vi "Excel文件读写.vi"(0 "选项":T1, 1 "sheet name":string="ASDE", 2 "列首名称":string[](array[string]) caption="列首", 3 "表格":string[][](table), 4 "单个结果":bool[][](array[boolean]), 5 "error in":errorcluster caption="错误输入（无错误）", 6 "Path":path=path "D:/123.xls") -> (14 "表格操作正常":bool, 15 "data":string[][](table), 19 "error out":errorcluster caption="错误输出")   [LabVIEW 2014]
uses:
  <vilib>/addons/_office/excel.llb/Excel Get Data ([str]).vi
  <vilib>/Utility/NIReport.llb/Append Text Table to Report (wrap).vi
  <vilib>/Utility/NIReport.llb/NI_report.lvclass
  <vilib>/Utility/NIReport.llb/Excel/NI_Excel.lvclass
  <vilib>/addons/_office/NI_ReportGenerationToolkit.lvlib
panel:
  out "error out 2":errorcluster caption="error out"
  in  "Cpk计算数量":i32
  out "Path 2":path
  out "结束行":cluster{"row":i32, "column":i32}
  out "起始":cluster{i32, i32}
  out "position (Excel)":cluster{"row":i32, "column":i32}
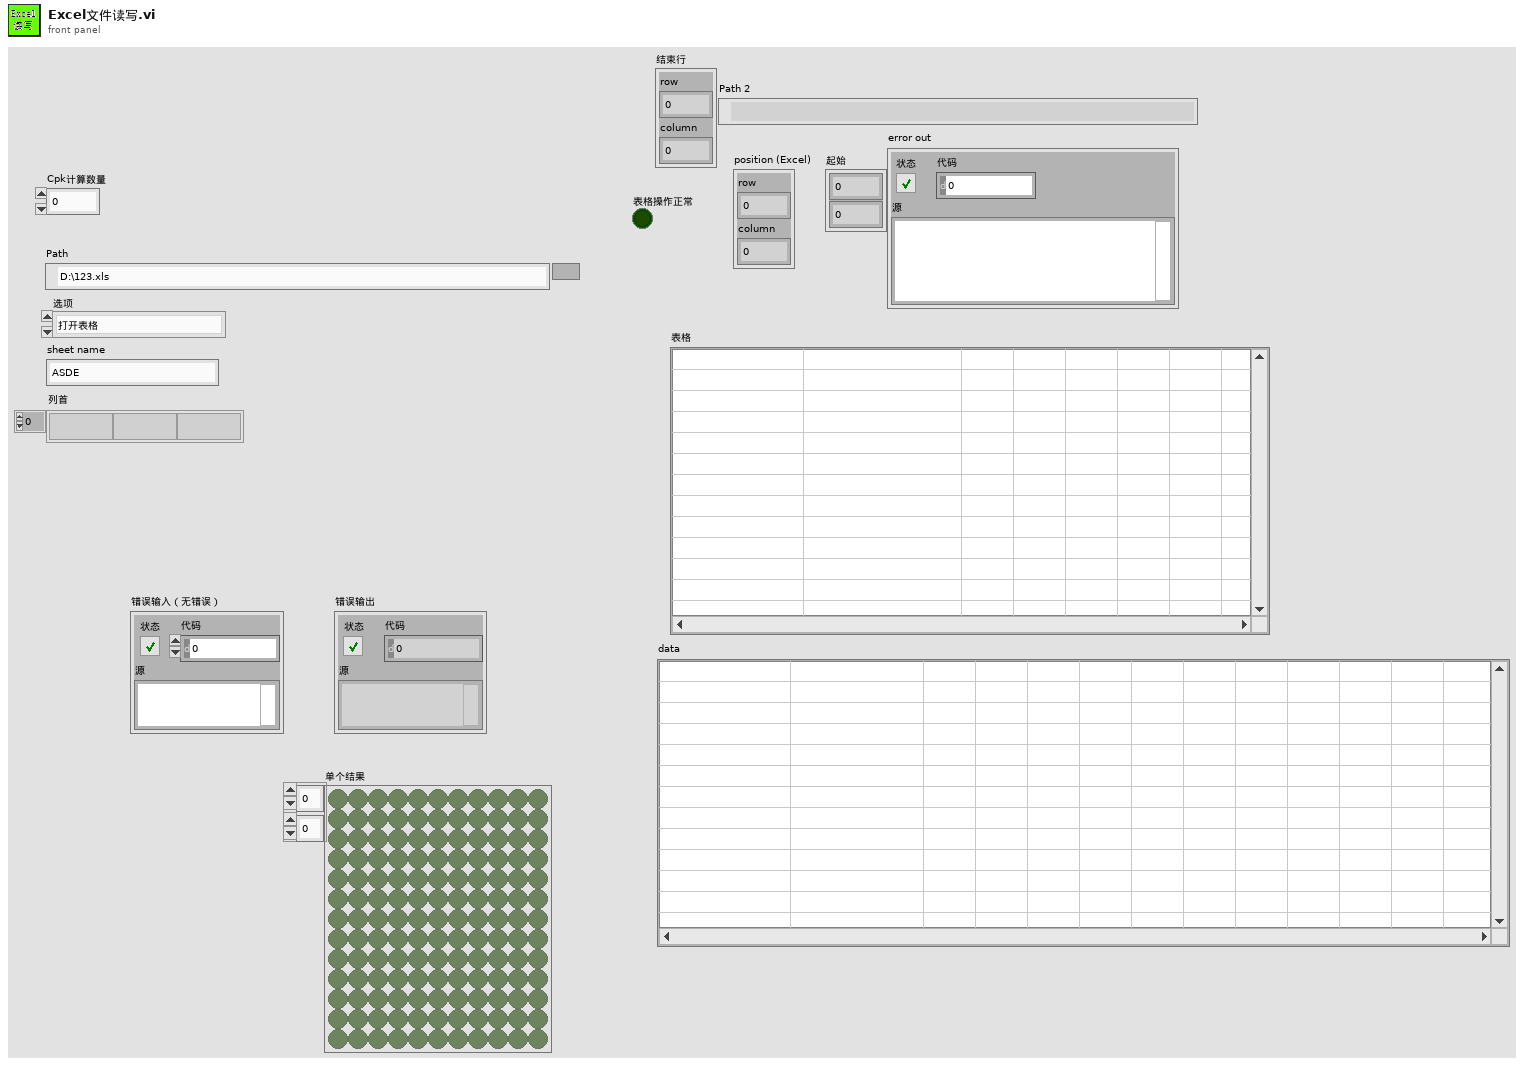
[diagram p1: front panel]
types:
  T1 = typedef "控件-Excel读写选项.ctl" = enum16{"打开表格", "新增sheet", "读取sheet指定位置数据", "读取sheet整个数据", "写入sheet整个数据", "写表头", "数据存到本机", "表格是否开启状态", "关闭表格"}
  T2 = enum16{"maximized", "minimized", "normal", "no change"}
  T3 = enum16{"Standard Report", "HTML", "Word", "Excel"}
  T4 = cluster{"position (Excel)":cluster{"row":i32, "column":i32}, "name (Excel)":string, "bookmark (Word)":string}
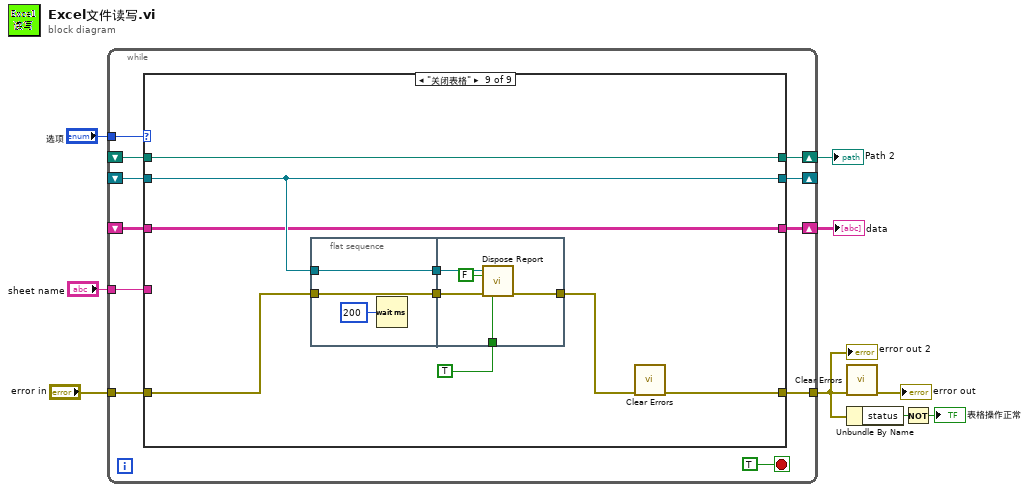
[diagram p0: block diagram]
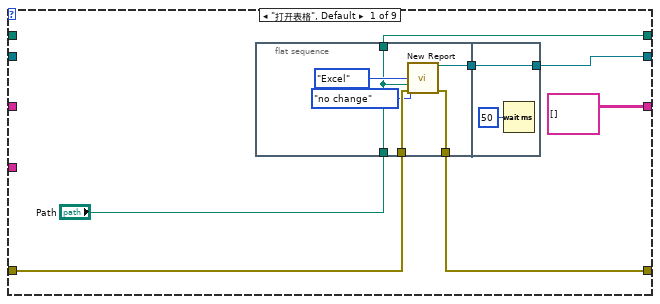
[diagram p2: hidden frame]
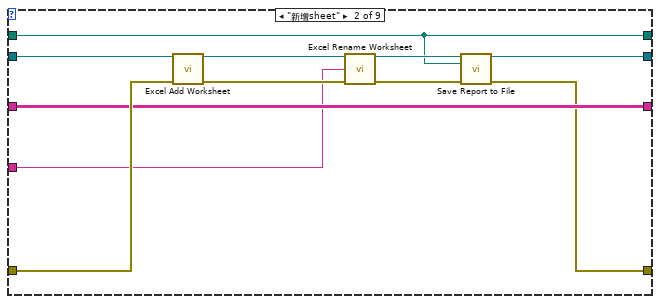
[diagram p3: hidden frame]
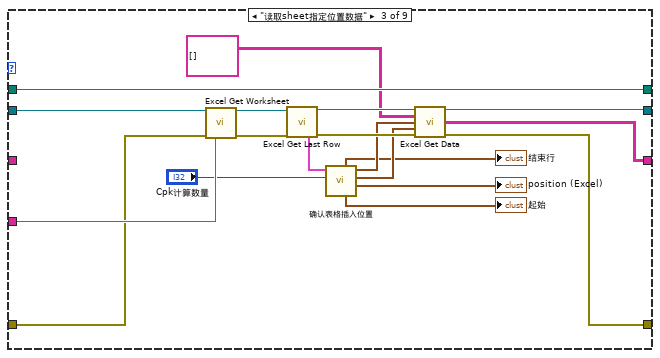
[diagram p4: hidden frame]
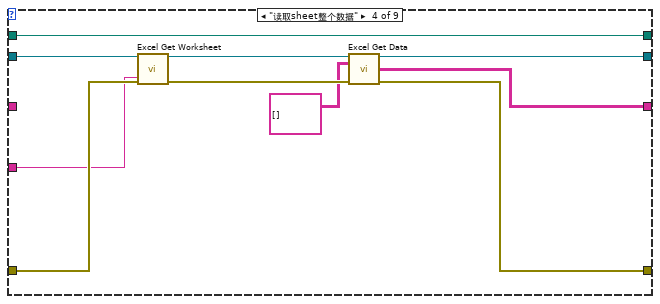
[diagram p5: hidden frame]
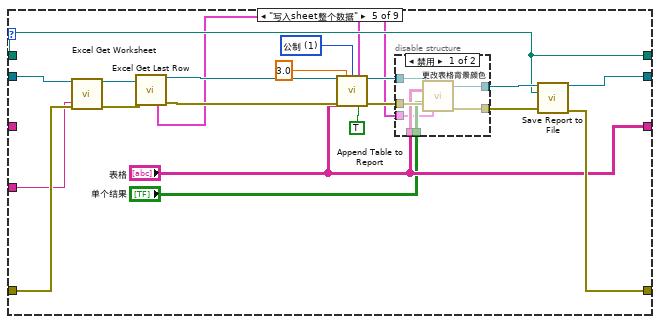
[diagram p6: hidden frame]
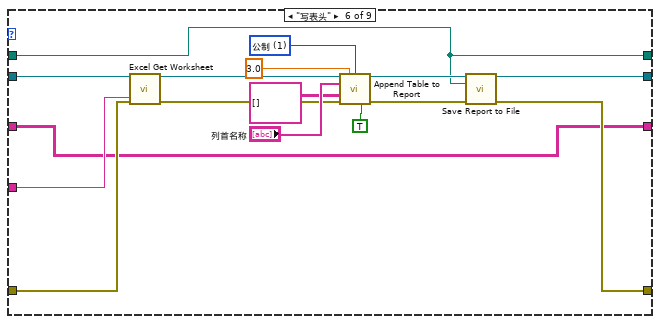
[diagram p8: hidden frame]
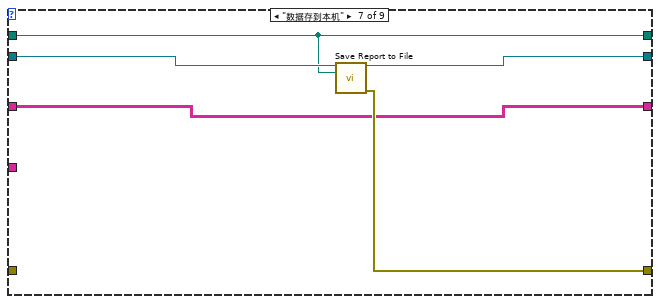
[diagram p9: hidden frame]
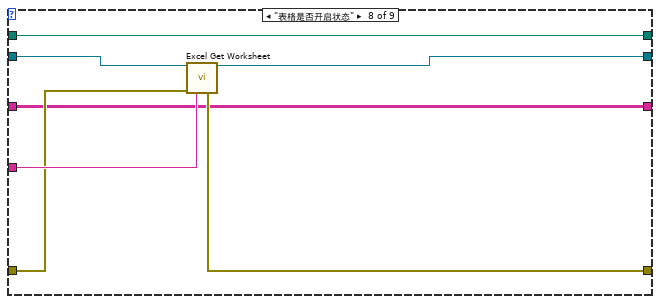
[diagram p10: hidden frame]
diagram:
  n1 = while {
    tunnel: "选项" -> [w19]
    shift-right: [w18] -> _
    shift-left: _ -> [w17]
    tunnel: "error in" -> [w16]
    tunnel: [w15] -> w4
    shift-right: [w14] -> w7
    shift-left: _ -> [w13]
    tunnel: "sheet name" -> [w12]
    shift-right: [w10] -> w1
    shift-left: _ -> [w11]
    stop <- TRUE stop-if-true
    n2 = case shown="\"关闭表格\"" w19 {
      tunnel: [w27 w39 w64 w73 w95 w115 w124 w128 w140] -> w18
      tunnel: w17 -> [_ w45 w56 w75 w90 w112 w125 w132 w140]
      tunnel: w16 -> [w26 w44 w57 w70 w89 w108 _ w130 w141]
      tunnel: [w25 w37 w65 w71 w94 w107 w123 w129 w136] -> w15
      tunnel: [string[][] [] ("data") w42 w63 w68 "表格" w105 w122 w126 w139] -> w14
      tunnel: w13 -> [_ w42 _ _ _ w105 w122 w126 w139]
      tunnel: w12 -> [_ w41 w58 w67 w88 w109 _ w131 _]
      tunnel: w11 -> [_ w36 w62 w66 w83 w110 w121 w127 w135]
      tunnel: [w22 w36 w62 w66 w83 w110 w121 w127 w135] -> w10
      frame "打开表格", Default {
        n3 = flat-sequence {
          tunnel: w26 -> [w32]
          tunnel: [w31] -> w25
          tunnel: "Path" -> [w28]
          tunnel: [w33] -> w23
          tunnel: [w28] -> w22
          tunnel: [w35] -> w27
          tunnel: w23 -> [w35]
          frame #0 {
            n4 = call <vilib>:"New Report.vi"("window state (normal)"=T2."no change", "report type"=T3."Excel", "template (empty)"=w28, "error in (no error)"=w32) -> ("report out"=w33:refnum<class "NI_report.lvclass">, "error out"=w31:errorcluster)  [unwired: 10 in]
          }
          frame #1 {
            n5 = Wait (ms)(milliseconds to wait=u32 50 ("等待时间（毫秒）")) -> ()  [unwired: 1 out]
          }
        }
      }
      frame "新增sheet" {
        n6 = call <vilib>:"Excel Add Worksheet.vi"("report in"=w45, "error in (no error)"=w44) -> ("report out"=w46:refnum<class "NI_report.lvclass">, "error out"=w43:errorcluster)  [unwired: 12 in]
        n7 = call <vilib>:"Excel Rename Worksheet.vi"("report in"=w46, "worksheet name (\"\")"=w41, "error in (no error)"=w43) -> ("report out"=w40:refnum<class "NI_report.lvclass">, "error out"=w38:errorcluster)  [unwired: 11 in]
        n8 = call-dynamic "Save Report to File.vi"("report in"=w40, "report file path"=w36, "error in (no error)"=w38) -> ("report out"=w39:refnum<class "NI_report.lvclass">, "error out"=w37:errorcluster)  [unwired: 11 in]
      }
      frame "读取sheet指定位置数据" {
        n9 = call <vilib>:"Excel Get Worksheet.vi"("report in"=w56, "error in (no error)"=w57, "name (\"\")"=w58) -> ("report out"=w55:refnum<class "NI_report.lvclass">, "error out"=w54:errorcluster)  [unwired: 11 in]
        n10 = call <vilib>:"Excel Get Last Row.vi"("report in"=w55, "error in (no error)"=w54) -> ("report out"=w61:refnum<class "NI_report.lvclass">, "MS Office parameters out"=w60:T4, "error out"=w59:errorcluster)  [unwired: 11 in]
        n11 = call "确认表格插入位置.vi"("Cpk计算数量"="Cpk计算数量", "MS Office parameters out"=w60) -> ("position (Excel)"=→"position (Excel)":cluster{"row":i32, "column":i32}, "簇"=w51:cluster{"row":i32, i32}, "簇 2"=w52:cluster{"f":i32, i32}, "起始"=→"起始":cluster{i32, i32}, "结束行"=→"结束行":cluster{"row":i32, "column":i32})  [unwired: 5 in]
        n12 = call-poly <vilib>:"Excel Get Data.vi"("report in"=w61, "data type"=string[][] [], "start (-1, -1)"=w52, "end (-1, -1)"=w51, "error in (no error)"=w59) -> ("report out"=w64:refnum<class "NI_report.lvclass">, "data"=w63:string[][], "error out"=w65:errorcluster)  [unwired: 8 in]
      }
      frame "读取sheet整个数据" {
        n13 = call <vilib>:"Excel Get Worksheet.vi"("report in"=w75, "error in (no error)"=w70, "name (\"\")"=w67) -> ("report out"=w74:refnum<class "NI_report.lvclass">, "error out"=w72:errorcluster)  [unwired: 11 in]
        n14 = call-poly <vilib>:"Excel Get Data.vi"("report in"=w74, "data type"=string[][] [], "error in (no error)"=w72) -> ("report out"=w73:refnum<class "NI_report.lvclass">, "data"=w68:string[][], "error out"=w71:errorcluster)  [unwired: 10 in]
      }
      frame "写入sheet整个数据" {
        w93 = u16 1 items=["US", "公制", "默认"] ("measurement system")
        n15 = call <vilib>:"Excel Get Worksheet.vi"("report in"=w90, "error in (no error)"=w89, "name (\"\")"=w88) -> ("report out"=w82:refnum<class "NI_report.lvclass">, "error out"=w81:errorcluster)  [unwired: 11 in]
        n16 = call <vilib>:"Excel Get Last Row.vi"("report in"=w82, "error in (no error)"=w81) -> ("report out"=w79:refnum<class "NI_report.lvclass">, "MS Office parameters out"=w76:T4, "error out"=w80:errorcluster)  [unwired: 11 in]
        n17 = call-poly <vilib>:"Append Table to Report.vi"("report in"=w79, "column width (1)"=3.0, "measurement system"=w93, "MS Office parameters"=w76, "text data"="表格", "error in (no error)"=w80, "show grid lines (YES)"=TRUE) -> ("report out"=w87:refnum<class "NI_report.lvclass">, "error out"=w85:errorcluster)  [unwired: 5 in, 2 out]
        n18 = disable-structure shown="禁用" {
          disable-tunnel: w87 -> [w102 w104]
          disable-tunnel: [w101 w103] -> w86
          disable-tunnel: w85 -> [w100 w103]
          disable-tunnel: [w99 w104] -> w84
          disable-tunnel: "表格" -> [w98 _]
          disable-tunnel: "单个结果" -> [w97 _]
          disable-tunnel: w76 -> [w96 _]
          frame Disabled {
            n19 = call "更改表格背景颜色.vi"("NI_report输入"=w102, "表格"=w98, "单个结果"=w97, "错误输入（无错误）"=w100, "MS Office parameters out"=w96) -> ("NI_report输出"=w99:refnum<class "NI_report.lvclass">, "错误输出"=w101:errorcluster)  [unwired: 9 in]
          }
          frame Enabled {
          }
        }
        n20 = call-dynamic "Save Report to File.vi"("report in"=w84, "report file path"=w83, "error in (no error)"=w86) -> ("report out"=w95:refnum<class "NI_report.lvclass">, "error out"=w94:errorcluster)  [unwired: 11 in]
      }
      frame "写表头" {
        w120 = u16 1 items=["US", "公制", "默认"] ("measurement system")
        n21 = call <vilib>:"Excel Get Worksheet.vi"("report in"=w112, "error in (no error)"=w108, "name (\"\")"=w109) -> ("report out"=w111:refnum<class "NI_report.lvclass">, "error out"=w113:errorcluster)  [unwired: 11 in]
        n22 = call-poly <vilib>:"Append Table to Report.vi"("report in"=w111, "column width (1)"=3.0, "measurement system"=w120, "column headers"="列首名称", "text data"=string[][] [], "error in (no error)"=w113, "show grid lines (YES)"=TRUE) -> ("report out"=w117:refnum<class "NI_report.lvclass">, "error out"=w116:errorcluster)  [unwired: 5 in, 2 out]
        n23 = call-dynamic "Save Report to File.vi"("report in"=w117, "report file path"=w110, "error in (no error)"=w116) -> ("report out"=w115:refnum<class "NI_report.lvclass">, "error out"=w107:errorcluster)  [unwired: 11 in]
      }
      frame "数据存到本机" {
        n24 = call-dynamic "Save Report to File.vi"("report in"=w125, "report file path"=w121) -> ("report out"=w124:refnum<class "NI_report.lvclass">, "error out"=w123:errorcluster)  [unwired: 12 in]
      }
      frame "表格是否开启状态" {
        n25 = call <vilib>:"Excel Get Worksheet.vi"("report in"=w132, "error in (no error)"=w130, "name (\"\")"=w131) -> ("report out"=w128:refnum<class "NI_report.lvclass">, "error out"=w129:errorcluster)  [unwired: 11 in]
      }
      frame "关闭表格" {
        n26 = flat-sequence {
          tunnel: w140 -> [w143]
          tunnel: w141 -> [w144]
          tunnel: [w144] -> w134
          tunnel: [w143] -> w133
          tunnel: TRUE ("close report? (T)") -> [w147]
          tunnel: w134 -> [w149]
          tunnel: w133 -> [w148]
          tunnel: [w145] -> w137
          frame #0 {
            n27 = Wait (ms)(milliseconds to wait=u32 200 ("等待时间（毫秒）")) -> ()  [unwired: 1 out]
          }
          frame #1 {
            n28 = call-dynamic "Dispose Report.vi"("report in"=w148, "wait until printing completed? (T)"=FALSE, "error in (no error)"=w149, "close report? (T)"=w147) -> ("error out"=w145:errorcluster)  [unwired: 11 in]
          }
        }
        n29 = call <vilib>:"Clear Errors.vi"("error in (no error)"=w137) -> ("error out"=w136:errorcluster)  [unwired: 5 in, 1 out]
      }
    }
  }
  "data" <- w7
  "Path 2" <- w1
  "error out 2" <- w4
  n30 = call <vilib>:"Clear Errors.vi"("error in (no error)"=w4) -> ("error out"=→"error out":errorcluster)  [unwired: 5 in, 1 out]
  n31 = Unbundle By Name(w4) -> ("status"=w3:bool)
  n32 = Not(x=w3) -> (.not. x?=→"表格操作正常":bool)
